vi "251213_XY Stage Move.vi"(8 "error in (no error)":errorcluster, 9 "Step size (mm?)":dbl, 10 "Label.Text":string, 11 "Automation Refnum in":refnum<k7>) -> (0 "error out":errorcluster, 3 "Automation Refnum out":refnum<k7>)   [LabVIEW 2025]
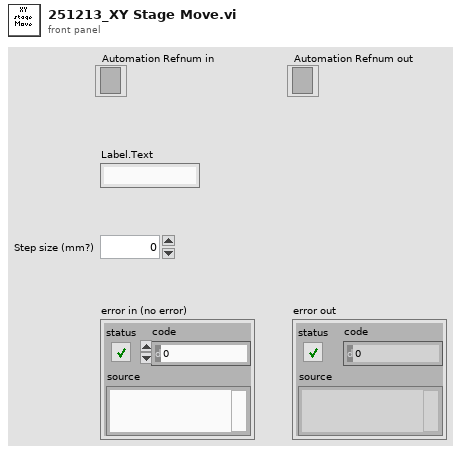
[diagram p1: front panel]
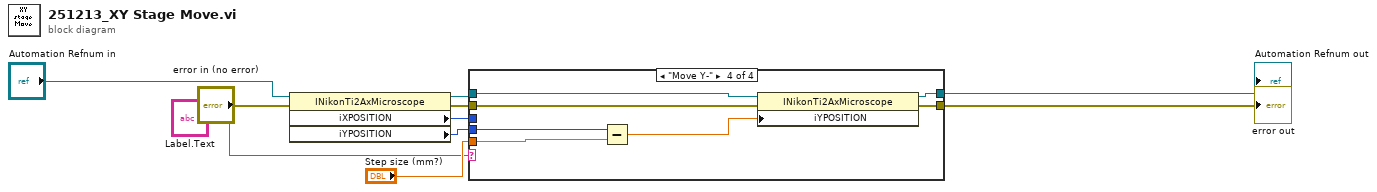
[diagram p0: block diagram]
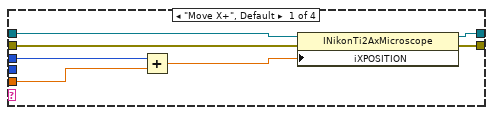
[diagram p2: hidden frame]
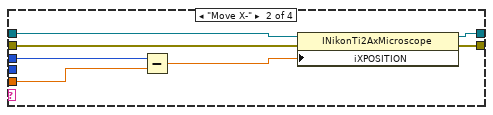
[diagram p3: hidden frame]
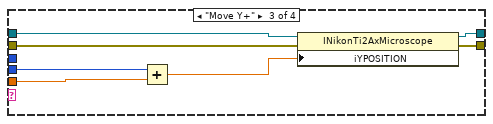
[diagram p4: hidden frame]
diagram:
  n1 = property class="INikonTi2AxMicroscope"(reference="Automation Refnum in", error in="error in (no error)") -> (reference out=w5:refnum<k7>, error out=w4:errorcluster, "iXPOSITION"=w6:i32, "iYPOSITION"=w7:i32)
  n2 = case shown="\"Move Y-\"" "Label.Text" {
    tunnel: w4 -> [w14 w23 w30 w35]
    tunnel: w5 -> [w13 w24 w31 w36]
    tunnel: w6 -> [w17 w22 _ _]
    tunnel: w7 -> [_ _ w29 w34]
    tunnel: "Step size (mm?)" -> [w16 w21 w28 w33]
    tunnel: [w12 w18 w25 w38] -> w9
    tunnel: [w11 w19 w26 w37] -> w10
    frame "Move X+", Default {
      n3 = Add(x=w17, y=w16) -> (x+y=w15:dbl)
      n4 = property class="INikonTi2AxMicroscope"(reference=w13, error in=w14, "iXPOSITION"=w15) -> (reference out=w12:refnum<k7>, error out=w11:errorcluster)
    }
    frame "Move X-" {
      n5 = Subtract(x=w22, y=w21) -> (x-y=w20:dbl)
      n6 = property class="INikonTi2AxMicroscope"(reference=w24, error in=w23, "iXPOSITION"=w20) -> (reference out=w18:refnum<k7>, error out=w19:errorcluster)
    }
    frame "Move Y+" {
      n7 = Add(x=w29, y=w28) -> (x+y=w27:dbl)
      n8 = property class="INikonTi2AxMicroscope"(reference=w31, error in=w30, "iYPOSITION"=w27) -> (reference out=w25:refnum<k7>, error out=w26:errorcluster)
    }
    frame "Move Y-" {
      n9 = Subtract(x=w34, y=w33) -> (x-y=w32:dbl)
      n10 = property class="INikonTi2AxMicroscope"(reference=w36, error in=w35, "iYPOSITION"=w32) -> (reference out=w38:refnum<k7>, error out=w37:errorcluster)
    }
  }
  "error out" <- w10
  "Automation Refnum out" <- w9
